vi "5207_Set_Frequency.vi"(2 "error in (no error)":errorcluster, 3 "Frequency (choose >=100)":i32=100 min=100 max=200000, 4 "VISA resource name":refnum<visa-resource-name>) -> (0 "error out":errorcluster, 1 "VISA resource name out":refnum<visa-resource-name>)   [LabVIEW 2015]
panel:
  out "write buffer":string
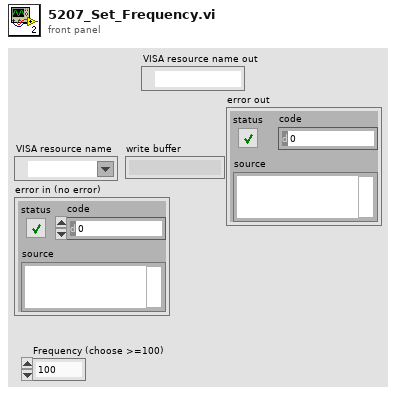
[diagram p1: front panel]
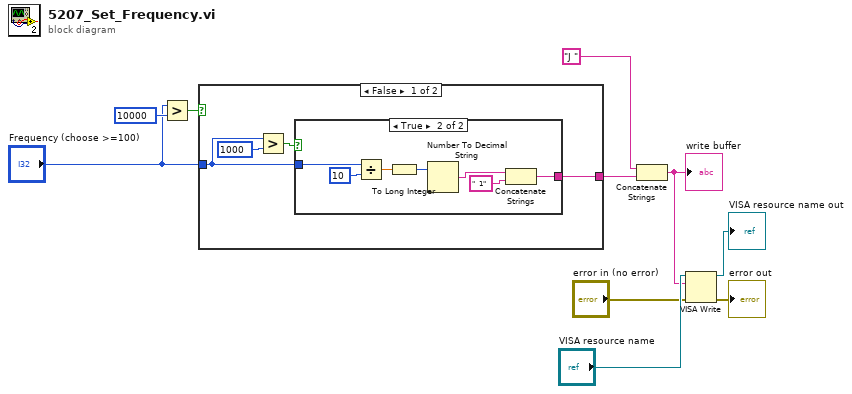
[diagram p0: block diagram]
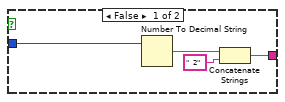
[diagram p2: hidden frame]
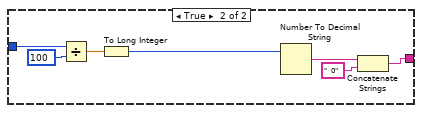
[diagram p3: hidden frame]
diagram:
  n1 = Greater?(x="Frequency (choose >=100)", y=10000) -> (0:w7:bool)
  n2 = case shown="False" w7 {
    tunnel: "Frequency (choose >=100)" -> [w12 w29]
    tunnel: [w11 w26] -> w5
    frame False {
      n3 = Greater?(x=w12, y=1000) -> (0:w13:bool)
      n4 = case shown="True" w13 {
        tunnel: w12 -> [w16 w20]
        tunnel: [w15 w19] -> w11
        frame False {
          n5 = Number To Decimal String(number=w16) -> (decimal integer string=w18:string)  [unwired: 1 in]
          n6 = Concatenate Strings(w18, "  2" ("string")) -> (w15:string)
        }
        frame True {
          n7 = Divide(x=w20, y=10) -> (x/y=w23:dbl)
          n8 = To Long Integer(number=w23) -> (32bit integer=w24:i32)
          n9 = Number To Decimal String(number=w24) -> (decimal integer string=w22:string)  [unwired: 1 in]
          n10 = Concatenate Strings(w22, "  1" ("string")) -> (w19:string)
        }
      }
    }
    frame True {
      n11 = Divide(x=w29, y=100) -> (x/y=w30:dbl)
      n12 = To Long Integer(number=w30) -> (32bit integer=w31:i32)
      n13 = Number To Decimal String(number=w31) -> (decimal integer string=w28:string)  [unwired: 1 in]
      n14 = Concatenate Strings(w28, "  0" ("string")) -> (w26:string)
    }
  }
  n15 = Concatenate Strings("J " ("string"), w5) -> (w4:string)
  "write buffer" <- w4
  n16 = VISA Write(VISA resource name="VISA resource name", write buffer=w4, error in (no error)="error in (no error)") -> (VISA resource name out=→"VISA resource name out":refnum<visa-resource-name>, error out=→"error out":errorcluster)  [unwired: 1 out]
